vi "HTML Report Image Attributes.vi"(5 "alignment (default)":T1, 6 "alt - alternative string":string) -> (2 "attributes out":string)   [LabVIEW 2020, in "NI_ReportGenerationCore.lvlib"]
doc: "Constructs image attributes for an image or image button tag <IMG,INPUT>."
uses:
  NI_ReportGenerationCore.lvlib
  HTML Report Image Alignment.ctl
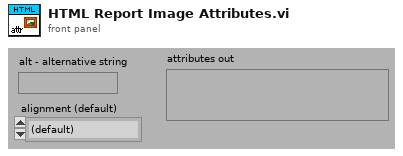
[diagram p1: front panel]
types:
  T1 = typedef "NI_ReportGenerationCore.lvlib/HTML Report Image Alignment.ctl" = enum16{"(default)", "LEFT", "RIGHT", "TOP", "TEXTTOP", "MIDDLE", "ABSMIDDLE", "BASELINE", "BOTTOM", "ABSBOTTOM"}
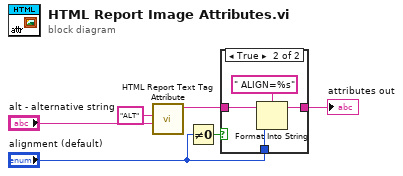
[diagram p0: block diagram]
diagram:
  n1 = call "HTML Report Text Tag Attribute.vi"("value"="alt - alternative string", "label"="ALT") -> ("tag attributes out"=w3:string)  [unwired: 2 in, 3 out]
  n2 = Not Equal To 0?(x="alignment (default)") -> (x != 0?=w6:bool)
  n3 = case shown="True" w6 {
    tunnel: w3 -> [w7 w9]
    tunnel: [w7 w8] -> w1
    tunnel: "alignment (default)" -> [_ w11]
    frame False {
    }
    frame True {
      n4 = Format Into String(format string=" ALIGN=%s", initial string=w9, w11) -> (resulting string=w8:string)  [unwired: 1 in, 1 out]
    }
  }
  "attributes out" <- w1
